vi "Fan Control VI.vi"() -> ()   [LabVIEW 2025]
doc: "This example demonstrates how to continuously read back the number of digital edges that have been counted by a counter input.\n\nFor instructions on how to connect your signals to the DAQ device, refer to your device documentation."
uses:
  <resource>/objmgr/daqmx.rc
  <vilib>/Utility/error.llb/DialogType.ctl
  <vilib>/DAQmx/read.llb/DAQmx Read (Counter U32 1Chan 1Samp).vi
  <vilib>/DAQmx/create/channels.llb/DAQmx Create Channel (CI-Count Edges).vi
  <vilib>/DAQmx/create/channels.llb/DAQmx Create Channel (CO-Pulse Generation-Frequency).vi
  <vilib>/DAQmx/configure/timing.llb/DAQmx Timing (Implicit).vi
  <vilib>/DAQmx/write.llb/DAQmx Write (Counter Frequency 1Chan 1Samp).vi
panel:
  in  "Type of Fan":u16(ring) items=["San Ace 80 12V 0.48A", "Orion 24V 1.7A", "San Ace 140 24V 2.3A"]
  in  "Duty Cycle 2":dbl(slide)=0.5 min=0.01 max=0.99 scale=0.0..1.0 scale format="%#_5g"
  in  "Output Terminal 2":tag="/Dev1/PFI12"
  in  "PWM Control 2":tag="Dev1/ctr0"
  in  "Active Edge 3":i32(ring)=10171 items=["Rising"=10280, "Falling"=10171]
  in  "Input Terminal 3":tag="PFI8"
  in  "RPM Counter 3":tag="Dev1/ctr0"
  out "Current RPM 3":u32
  out "Fan 3":dbl(graph)
  in  "Duty Cycle":dbl(slide)=0.5 min=0.01 max=0.99 scale=0.0..1.0
  in  "Output Terminal":tag="/Dev1/PFI12"
  in  "PWM Control":tag="Dev1/ctr0"
  in  "Master Stop":bool
  in  "Active Edge 2":i32(ring)=10171 items=["Rising"=10280, "Falling"=10171]
  in  "Input Terminal 2":tag="PFI8"
  in  "RPM Counter 2":tag="Dev1/ctr0"
  out "Current RPM 2":u32
  out "Fan 2":dbl(graph)
  out "Fan 1":dbl(graph)
  out "Current RPM":u32
  in  "Active Edge":i32(ring)=10171 items=["Rising"=10280, "Falling"=10171]
  in  "Input Terminal":tag="PFI8"
  in  "RPM Counter1":tag="Dev1/ctr0"
  # "Current RPM"
  # "Channel Settings"
  # "RPM Graphs"
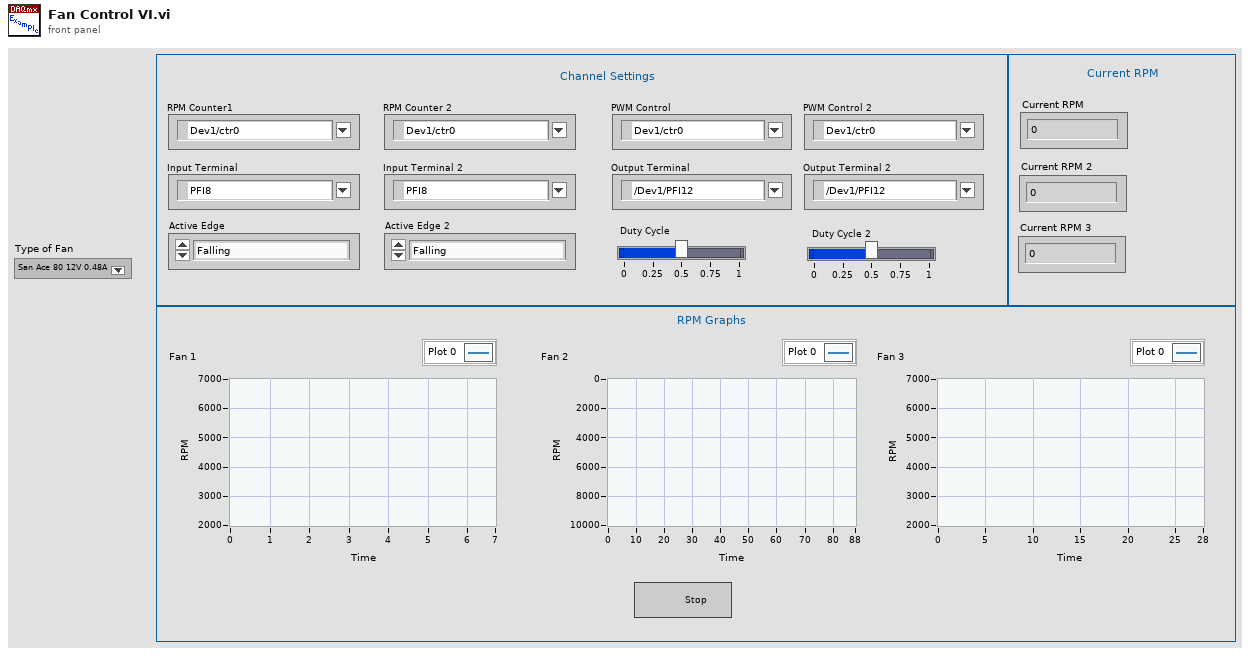
[diagram p1: front panel]
types:
  T1 = typedef "DialogType.ctl" = u16
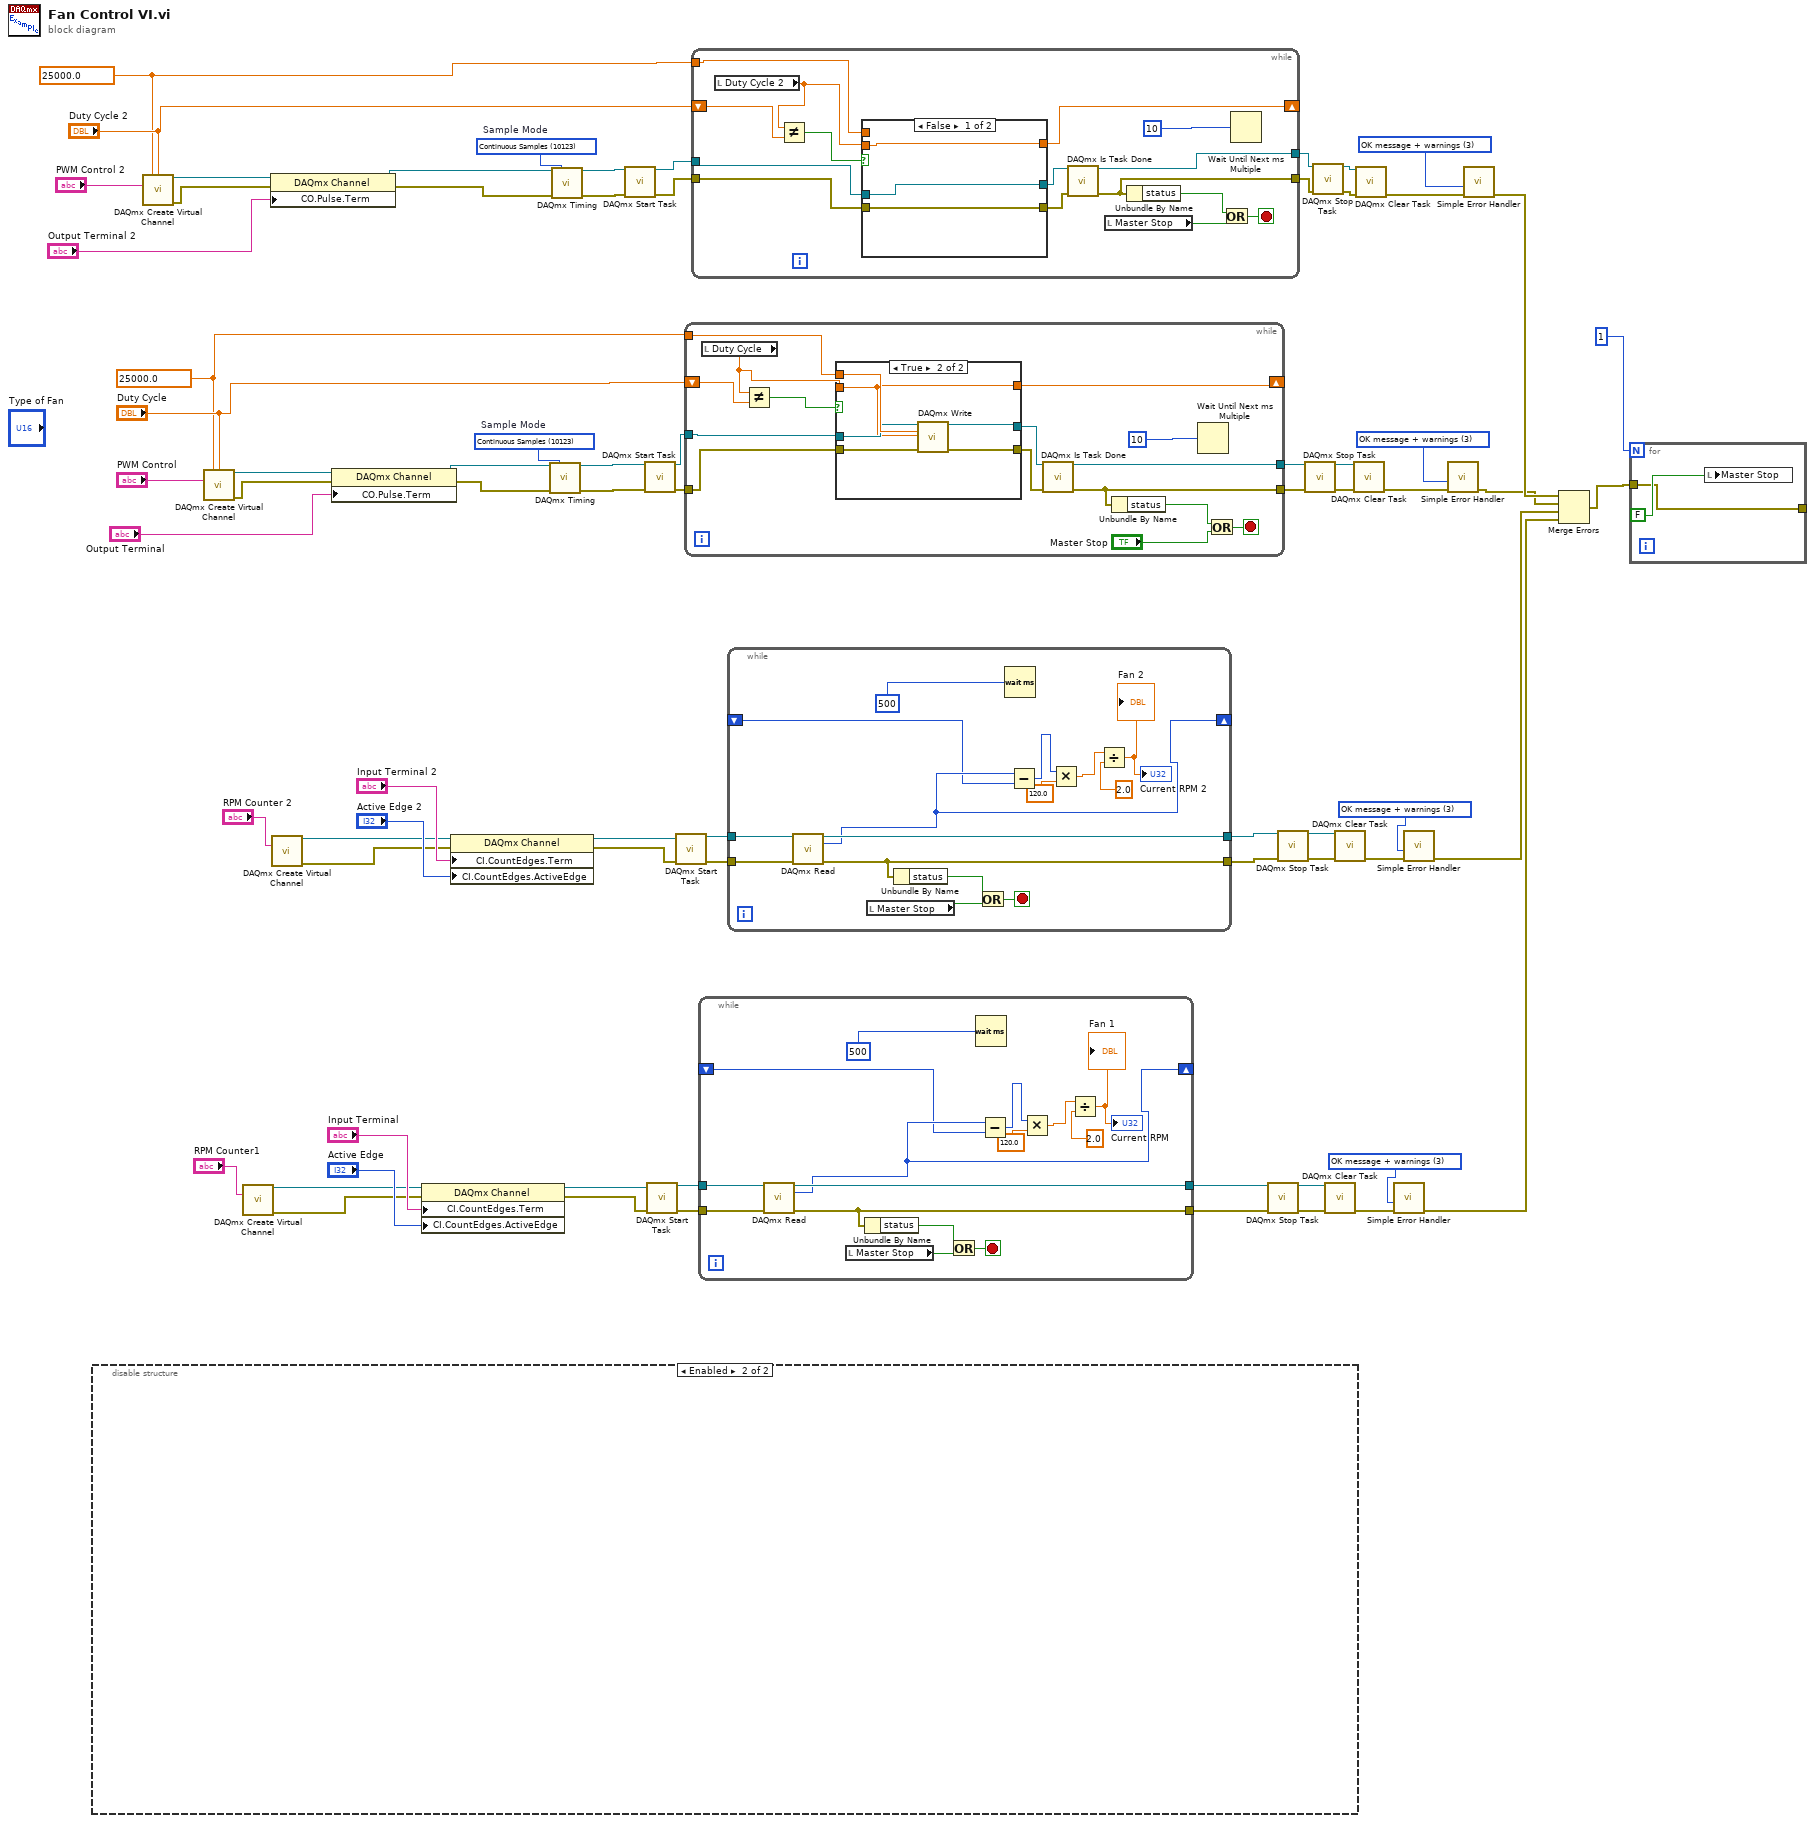
[diagram p0: block diagram]
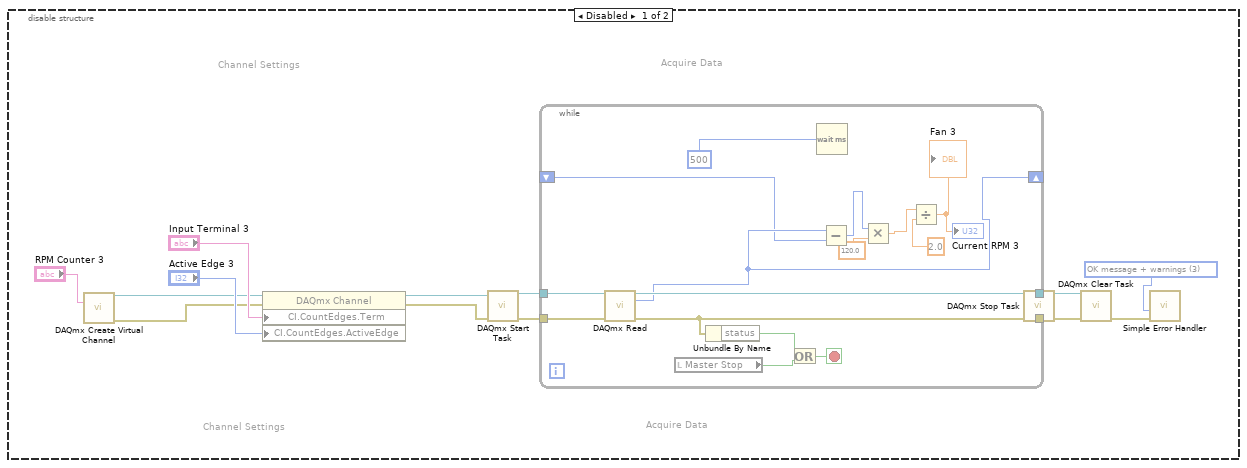
[diagram p2: hidden frame]
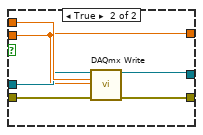
[diagram p3: hidden frame]
diagram:
  w3 = 25000.0 ("Frequency")
  w11 = T1 3 items=["no dialog", "OK message", "continue or stop message", "OK message + warnings", "continue/stop + warnings"] ("type of dialog (OK msg:1)")
  w27 = 10123 items=["Finite Samples"=10178, "Continuous Samples"=10123, "Hardware Timed Single Point"=12522]  # Sample Mode
  w1 = 25000.0 ("Frequency")
  w28 = T1 3 items=["no dialog", "OK message", "continue or stop message", "OK message + warnings", "continue/stop + warnings"] ("type of dialog (OK msg:1)")
  w44 = 10123 items=["Finite Samples"=10178, "Continuous Samples"=10123, "Hardware Timed Single Point"=12522]  # Sample Mode
  w46 = T1 3 items=["no dialog", "OK message", "continue or stop message", "OK message + warnings", "continue/stop + warnings"] ("type of dialog (OK msg:1)")
  w60 = T1 3 items=["no dialog", "OK message", "continue or stop message", "OK message + warnings", "continue/stop + warnings"] ("type of dialog (OK msg:1)")
  n1 = disable-structure shown="Enabled" {
    frame Disabled {
      w75 = T1 3 items=["no dialog", "OK message", "continue or stop message", "OK message + warnings", "continue/stop + warnings"] ("type of dialog (OK msg:1)")
      # "Acquire Data"
      # "Channel Settings"
      # "Acquire Data"
      # "Channel Settings"
      n2 = call-poly <vilib>:"DAQmx Create Virtual Channel.vi"("counter"="RPM Counter 3") -> ("task out"=w83:refnum<k21>, "error out"=w82:errorcluster)  [unwired: 13 in]
      n3 = property class="DAQmx Channel"(reference=w83, error in=w82, "CI.CountEdges.Term"="Input Terminal 3", "CI.CountEdges.ActiveEdge"="Active Edge 3") -> (reference out=w80:refnum<k21>, error out=w81:errorcluster)
      n4 = call <vilib>:"DAQmx Start Task.vi"("task/channels in"=w80, "error in"=w81) -> ("task out"=w87:refnum<k21>, "error out"=w86:errorcluster)  [unwired: 12 in]
      n5 = while {
        tunnel: w87 -> [w104]
        tunnel: w86 -> [w103]
        tunnel: [w100] -> w78
        tunnel: [w101] -> w79
        shift-right: [w95] -> _
        shift-left: _ -> [w92]
        stop <- w102 stop-if-true
        n6 = call-poly <vilib>:"DAQmx Read.vi"("task/channels in"=w104, "error in"=w103) -> ("task out"=w101:refnum<k21>, "data"=w95:u32, "error out"=w100:errorcluster)  [unwired: 11 in]
        n7 = local read "Master Stop"() -> (w90:bool)
        n8 = Unbundle By Name(w100) -> ("status"=w99:bool)
        n9 = Or(x=w99, y=w90) -> (x .or. y?=w102:bool)
        n10 = Wait (ms)(milliseconds to wait=u32 500 ("Loop Time (ms)")) -> ()  [unwired: 1 out]
        n11 = Subtract(x=w95, y=w92) -> (x-y=w96:u32)
        n12 = Multiply(x=w96, y=120.0) -> (x*y=w94:dbl)
        n13 = Divide(x=w94, y=2.0) -> (x/y=→"Current RPM 3" →"Fan 3":dbl)
      }
      n14 = call <vilib>:"DAQmx Stop Task.vi"("task/channels in"=w79, "error in"=w78) -> ("task out"=w76:refnum<k21>, "error out"=w77:errorcluster)  [unwired: 12 in]
      n15 = call <vilib>:"DAQmx Clear Task.vi"("task in"=w76, "error in"=w77) -> ("error out"=w85:errorcluster)  [unwired: 13 in]
      n16 = call <vilib>:"Simple Error Handler.vi"("type of dialog (OK msg:1)"=w75, "error in (no error)"=w85) -> ()  [unwired: 3 in, 5 out]
    }
    frame Enabled {
    }
  }
  n17 = call-poly <vilib>:"DAQmx Create Virtual Channel.vi"("frequency"=w3, "duty cycle"="Duty Cycle 2", "counter"="PWM Control 2") -> ("task out"=w20:refnum<k21>, "error out"=w19:errorcluster)  [unwired: 11 in]
  n18 = call-poly <vilib>:"DAQmx Create Virtual Channel.vi"("frequency"=w1, "duty cycle"="Duty Cycle", "counter"="PWM Control") -> ("task out"=w37:refnum<k21>, "error out"=w36:errorcluster)  [unwired: 11 in]
  n19 = call-poly <vilib>:"DAQmx Create Virtual Channel.vi"("counter"="RPM Counter1") -> ("task out"=w68:refnum<k21>, "error out"=w67:errorcluster)  [unwired: 13 in]
  n20 = property class="DAQmx Channel"(reference=w20, error in=w19, "CO.Pulse.Term"="Output Terminal 2") -> (reference out=w16:refnum<k21>, error out=w17:errorcluster)
  n21 = call-poly <vilib>:"DAQmx Create Virtual Channel.vi"("counter"="RPM Counter 2") -> ("task out"=w54:refnum<k21>, "error out"=w53:errorcluster)  [unwired: 13 in]
  n22 = property class="DAQmx Channel"(reference=w37, error in=w36, "CO.Pulse.Term"="Output Terminal") -> (reference out=w33:refnum<k21>, error out=w34:errorcluster)
  n23 = property class="DAQmx Channel"(reference=w68, error in=w67, "CI.CountEdges.Term"="Input Terminal", "CI.CountEdges.ActiveEdge"="Active Edge") -> (reference out=w65:refnum<k21>, error out=w66:errorcluster)
  n24 = property class="DAQmx Channel"(reference=w54, error in=w53, "CI.CountEdges.Term"="Input Terminal 2", "CI.CountEdges.ActiveEdge"="Active Edge 2") -> (reference out=w51:refnum<k21>, error out=w52:errorcluster)
  n25 = call-poly <vilib>:"DAQmx Timing.vi"("task/channels in"=w33, "sample mode"=w44, "error in"=w34) -> ("task out"=w39:refnum<k21>, "error out"=w38:errorcluster)  [unwired: 11 in]
  n26 = call-poly <vilib>:"DAQmx Timing.vi"("task/channels in"=w16, "sample mode"=w27, "error in"=w17) -> ("task out"=w22:refnum<k21>, "error out"=w21:errorcluster)  [unwired: 11 in]
  n27 = call <vilib>:"DAQmx Start Task.vi"("task/channels in"=w22, "error in"=w21) -> ("task out"=w26:refnum<k21>, "error out"=w25:errorcluster)  [unwired: 12 in]
  n28 = call <vilib>:"DAQmx Start Task.vi"("task/channels in"=w39, "error in"=w38) -> ("task out"=w43:refnum<k21>, "error out"=w42:errorcluster)  [unwired: 12 in]
  n29 = call <vilib>:"DAQmx Start Task.vi"("task/channels in"=w65, "error in"=w66) -> ("task out"=w72:refnum<k21>, "error out"=w71:errorcluster)  [unwired: 12 in]
  n30 = call <vilib>:"DAQmx Start Task.vi"("task/channels in"=w51, "error in"=w52) -> ("task out"=w57:refnum<k21>, "error out"=w56:errorcluster)  [unwired: 12 in]
  n31 = while {
    tunnel: w43 -> [w110]
    tunnel: w42 -> [w113]
    tunnel: [w117] -> w29
    tunnel: [w118] -> w30
    tunnel: w1 -> [w106]
    shift-right: [w105] -> _
    shift-left: "Duty Cycle" -> [w108]
    stop <- w119 stop-if-true
    n32 = local read "Duty Cycle"() -> (w107:dbl)
    n33 = Not Equal?(x=w107, y=w108) -> (x != y?=w109:bool)
    n34 = case shown="True" w109 {
      tunnel: [w121 w127] -> w112
      tunnel: w113 -> [w121 w128]
      tunnel: [w122 w124] -> w111
      tunnel: w110 -> [w122 w125]
      tunnel: w107 -> [w120 w123]
      tunnel: w106 -> [_ w126]
      tunnel: [w120 w123] -> w105
      frame False {
      }
      frame True {
        n35 = call-poly <vilib>:"DAQmx Write.vi"("task/channels in"=w125, "frequency"=w126, "duty cycle"=w123, "error in"=w128) -> ("task out"=w124:refnum<k21>, "error out"=w127:errorcluster)  [unwired: 9 in, 1 out]
      }
    }
    n36 = call <vilib>:"DAQmx Is Task Done.vi"("task/channels in"=w111, "error in"=w112) -> ("task out"=w118:refnum<k21>, "error out"=w117:errorcluster)  [unwired: 11 in, 1 out]
    n37 = Unbundle By Name(w117) -> ("status"=w116:bool)
    n38 = Wait Until Next ms Multiple(millisecond multiple=u32 10) -> ()  [unwired: 1 out]
    n39 = Or(x=w116, y="Master Stop") -> (x .or. y?=w119:bool)
  }
  n40 = while {
    tunnel: w26 -> [w134]
    tunnel: w25 -> [w136]
    tunnel: [w141] -> w12
    tunnel: [w142] -> w13
    tunnel: w3 -> [w130]
    shift-right: [w129] -> _
    shift-left: "Duty Cycle 2" -> [w133]
    stop <- w143 stop-if-true
    n41 = local read "Duty Cycle 2"() -> (w131:dbl)
    n42 = Not Equal?(x=w131, y=w133) -> (x != y?=w132:bool)
    n43 = case shown="False" w132 {
      tunnel: [w145 w151] -> w137
      tunnel: w136 -> [w145 w152]
      tunnel: [w146 w148] -> w135
      tunnel: w134 -> [w146 w149]
      tunnel: w131 -> [w144 w147]
      tunnel: w130 -> [_ w150]
      tunnel: [w144 w147] -> w129
      frame False {
      }
      frame True {
        n44 = call-poly <vilib>:"DAQmx Write.vi"("task/channels in"=w149, "frequency"=w150, "duty cycle"=w147, "error in"=w152) -> ("task out"=w148:refnum<k21>, "error out"=w151:errorcluster)  [unwired: 9 in, 1 out]
      }
    }
    n45 = call <vilib>:"DAQmx Is Task Done.vi"("task/channels in"=w135, "error in"=w137) -> ("task out"=w142:refnum<k21>, "error out"=w141:errorcluster)  [unwired: 11 in, 1 out]
    n46 = local read "Master Stop"() -> (w138:bool)
    n47 = Unbundle By Name(w141) -> ("status"=w140:bool)
    n48 = Or(x=w140, y=w138) -> (x .or. y?=w143:bool)
    n49 = Wait Until Next ms Multiple(millisecond multiple=u32 10) -> ()  [unwired: 1 out]
  }
  n50 = while {
    tunnel: w72 -> [w167]
    tunnel: w71 -> [w166]
    tunnel: [w163] -> w63
    tunnel: [w164] -> w64
    shift-right: [w158] -> _
    shift-left: _ -> [w155]
    stop <- w165 stop-if-true
    n51 = call-poly <vilib>:"DAQmx Read.vi"("task/channels in"=w167, "error in"=w166) -> ("task out"=w164:refnum<k21>, "data"=w158:u32, "error out"=w163:errorcluster)  [unwired: 11 in]
    n52 = local read "Master Stop"() -> (w153:bool)
    n53 = Unbundle By Name(w163) -> ("status"=w162:bool)
    n54 = Or(x=w162, y=w153) -> (x .or. y?=w165:bool)
    n55 = Wait (ms)(milliseconds to wait=u32 500 ("Loop Time (ms)")) -> ()  [unwired: 1 out]
    n56 = Subtract(x=w158, y=w155) -> (x-y=w159:u32)
    n57 = Multiply(x=w159, y=120.0) -> (x*y=w157:dbl)
    n58 = Divide(x=w157, y=2.0) -> (x/y=→"Current RPM" →"Fan 1":dbl)
  }
  n59 = while {
    tunnel: w57 -> [w182]
    tunnel: w56 -> [w181]
    tunnel: [w178] -> w49
    tunnel: [w179] -> w50
    shift-right: [w173] -> _
    shift-left: _ -> [w170]
    stop <- w180 stop-if-true
    n60 = call-poly <vilib>:"DAQmx Read.vi"("task/channels in"=w182, "error in"=w181) -> ("task out"=w179:refnum<k21>, "data"=w173:u32, "error out"=w178:errorcluster)  [unwired: 11 in]
    n61 = local read "Master Stop"() -> (w168:bool)
    n62 = Unbundle By Name(w178) -> ("status"=w177:bool)
    n63 = Or(x=w177, y=w168) -> (x .or. y?=w180:bool)
    n64 = Wait (ms)(milliseconds to wait=u32 500 ("Loop Time (ms) 2")) -> ()  [unwired: 1 out]
    n65 = Subtract(x=w173, y=w170) -> (x-y=w174:u32)
    n66 = Multiply(x=w174, y=120.0) -> (x*y=w172:dbl)
    n67 = Divide(x=w172, y=2.0) -> (x/y=→"Current RPM 2" →"Fan 2":dbl)
  }
  n68 = call <vilib>:"DAQmx Stop Task.vi"("task/channels in"=w64, "error in"=w63) -> ("task out"=w61:refnum<k21>, "error out"=w62:errorcluster)  [unwired: 12 in]
  n69 = call <vilib>:"DAQmx Stop Task.vi"("task/channels in"=w50, "error in"=w49) -> ("task out"=w47:refnum<k21>, "error out"=w48:errorcluster)  [unwired: 12 in]
  n70 = call <vilib>:"DAQmx Stop Task.vi"("task/channels in"=w30, "error in"=w29) -> ("task out"=w32:refnum<k21>, "error out"=w31:errorcluster)  [unwired: 12 in]
  n71 = call <vilib>:"DAQmx Stop Task.vi"("task/channels in"=w13, "error in"=w12) -> ("task out"=w15:refnum<k21>, "error out"=w14:errorcluster)  [unwired: 12 in]
  n72 = call <vilib>:"DAQmx Clear Task.vi"("task in"=w61, "error in"=w62) -> ("error out"=w70:errorcluster)  [unwired: 13 in]
  n73 = call <vilib>:"DAQmx Clear Task.vi"("task in"=w47, "error in"=w48) -> ("error out"=w55:errorcluster)  [unwired: 13 in]
  n74 = call <vilib>:"DAQmx Clear Task.vi"("task in"=w32, "error in"=w31) -> ("error out"=w41:errorcluster)  [unwired: 13 in]
  n75 = call <vilib>:"DAQmx Clear Task.vi"("task in"=w15, "error in"=w14) -> ("error out"=w24:errorcluster)  [unwired: 13 in]
  n76 = call <vilib>:"Simple Error Handler.vi"("type of dialog (OK msg:1)"=w60, "error in (no error)"=w70) -> ("error out"=w7:errorcluster)  [unwired: 3 in, 4 out]
  n77 = call <vilib>:"Simple Error Handler.vi"("type of dialog (OK msg:1)"=w46, "error in (no error)"=w55) -> ("error out"=w8:errorcluster)  [unwired: 3 in, 4 out]
  n78 = call <vilib>:"Simple Error Handler.vi"("type of dialog (OK msg:1)"=w28, "error in (no error)"=w41) -> ("error out"=w9:errorcluster)  [unwired: 3 in, 4 out]
  n79 = call <vilib>:"Simple Error Handler.vi"("type of dialog (OK msg:1)"=w11, "error in (no error)"=w24) -> ("error out"=w10:errorcluster)  [unwired: 3 in, 4 out]
  n80 = Merge Errors(w10, w9, w8, w7) -> (w6:errorcluster)
  n81 = for {
    N: 1 ("Numeric") -> [_]
    tunnel: w6 -> [w183]
    tunnel: [w183] -> _
    n82 = local write "Master Stop"(FALSE ("Master Stop  2")) -> ()
  }
